vi "Set Discovery Endpoint.vi"(8 "error in (no error)":errorcluster, 10 "Discovery Endpoint":T1, 11 "Cluster in":refnum<class "Cluster.lvclass">) -> (0 "error out":errorcluster, 3 "Cluster out":refnum<class "Cluster.lvclass">)   [LabVIEW 2020, in "VolatusConfig.lvlib" / "Cluster.lvclass"]
uses:
  Cluster.lvclass
  lv-cdm/CDM-Config/Config Element/Config Element.lvclass
  VolatusConfigElement/VolatusConfigElement.lvclass
  lv-cdm/CDM-Config/Value Type.ctl
  lv-cdm/CDM-Config/CDM-Config.lvlib
  C:/dev/lv20CE/relink/lv-volatus/VolatusConfig/VolatusConfigElement/VolatusConfigElement.lvclass
  C:/dev/lv20CE/relink/lv-volatus/VolatusConfig/Cluster/Cluster.lvclass
  Endpoint.ctl
  VolatusConfig.lvlib
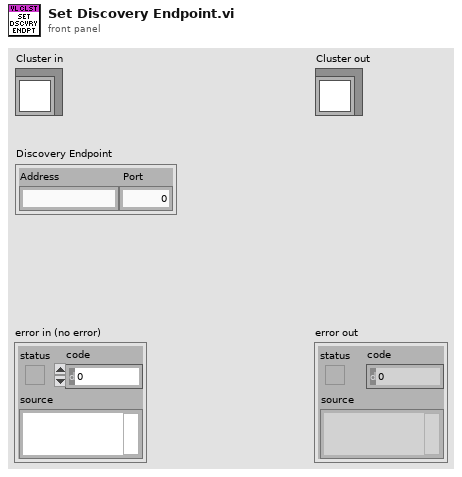
[diagram p1: front panel]
types:
  T1 = typedef "VolatusConfig.lvlib/Endpoint.ctl" = cluster{"Address":string, "Port":u16}
  T2 = typedef "CDM-Config.lvlib/Value Type.ctl" = enum16{"String", "Number", "Bool", "Object", "Array"}
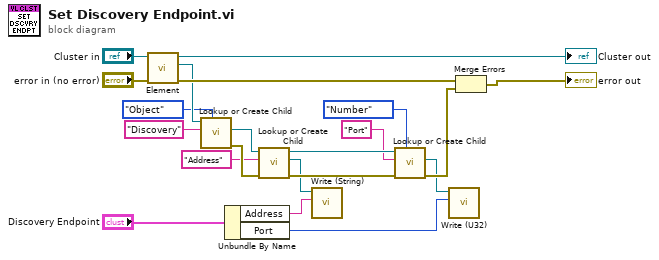
[diagram p0: block diagram]
diagram:
  n1 = call "Element.vi"("VolatusConfigElement in"="Cluster in") -> ("Element"=w15:refnum<class "Config Element.lvclass">, "VolatusConfigElement out"=→"Cluster out":refnum<class "Cluster.lvclass">)  [unwired: 9 in]
  n2 = call "Lookup or Create Child.vi"("Value Type (String)"=Value_Type."Object", "Name"="Discovery", "Config Element in"=w15) -> ("error out"=w19:errorcluster, "Child"=w12:refnum<class "Config Element.lvclass">)  [unwired: 5 in, 2 out]
  n3 = Unbundle By Name("Discovery Endpoint") -> ("Address"=w4:string, "Port"=w2:u16)
  n4 = call "Lookup or Create Child.vi"("error in (no error)"=w19, "Name"="Address", "Config Element in"=w12) -> ("error out"=w9:errorcluster, "Child"=w5:refnum<class "Config Element.lvclass">, "Config Element out"=w10:refnum<class "Config Element.lvclass">)  [unwired: 5 in, 1 out]
  n5 = call "Write (String).vi"("String Value"=w4, "Config Element in"=w5) -> ()  [unwired: 8 in, 2 out]
  n6 = call "Lookup or Create Child.vi"("Value Type (String)"=Value_Type."Number", "error in (no error)"=w9, "Name"="Port", "Config Element in"=w10) -> ("error out"=w20:errorcluster, "Child"=w3:refnum<class "Config Element.lvclass">)  [unwired: 4 in, 2 out]
  n7 = call "Write (U32).vi"("U32 Value"=w2, "Config Element in"=w3) -> ()  [unwired: 8 in, 2 out]
  n8 = Merge Errors("error in (no error)", w20) -> (→"error out":errorcluster)
